vi "Periodic Tasks.vi"(8 "error in":errorcluster) -> ()   [LabVIEW 2017]
doc: "This VI runs in parallel to other tasks. It can contain as many user-defined periodic loops as you need. These can carry out PID or other sorts of timed response."
uses:
  HuskieBoard.ctl
  Log Queue.ctl
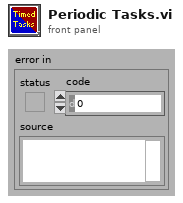
[diagram p1: front panel]
types:
  T1 = typedef "Log Queue.ctl" = enum16{"Log Queue"}
  T2 = typedef "HuskieBoard.ctl" = enum16{"HuskieBoard"}
  T3 = typedef "WPI_JoystickDevRef.ctl" = cluster{"Device":T4}
  T4 = typedef "WPI_JoystickDeviceEnum.ctl" = enum16{"USB 0", "USB 1", "USB 2", "USB 3", "USB 4", "USB 5"}
  T5 = typedef "WPI_RobotDriveDevRef.ctl" = cluster{"DevStatus":errorcluster, "Motors[]":T6[], "Square Inputs":bool, "Max Output":dbl}
  T6 = typedef "WPI_MotorControlDeviceRef.ctl" = cluster{"DeviceStatus":errorcluster, "Type":T7, "PWM":cluster{"PWM Channel":T8, "DeadBand":T9}, "CAN":cluster{"Device Number":u8, "SetOutput VI Ref":variant, "GetOutput VI Ref":variant, "Enable VI Ref":variant, "Disable VI Ref":variant, "Data":variant}, "Invert":bool, "DIO PWM":cluster{"PWM \"Enable\" Channel":T8, "DIOChannel":T10, "PWM Rate":dbl}}
  T7 = typedef "WPI_MotorControlType.ctl" = enum16{"PWM", "CAN", "DIO PWM"}
  T8 = typedef "FPGA_DIOPWMChannel.ctl" = enum8{"PWM 0", "PWM 1", "PWM 2", "PWM 3", "PWM 4", "PWM 5", "PWM 6", "PWM 7", "PWM 8", "PWM 9", "PWM MXP 0", "PWM MXP 1", "PWM MXP 2", "PWM MXP 3", "PWM MXP 4", "PWM MXP 5", "PWM MXP 6", "PWM MXP 7", "PWM MXP 8", "PWM MXP 9", "Invalid"}
  T9 = typedef "WPI_PWMDeadband.ctl" = cluster{"Name":string, "maxPositivePwm":i32, "minPositivePwm":i32, "centerPwm":i32, "maxNegativePwm":i32, "minNegativePwm":i32, "angularRange":u16}
  T10 = typedef "FPGA_DIOChannel.ctl" = enum8{"DIO 0", "DIO 1", "DIO 2", "DIO 3", "DIO 4", "DIO 5", "DIO 6", "DIO 7", "DIO 8", "DIO 9", "DIO MXP 0", "DIO MXP 1", "DIO MXP 2", "DIO MXP 3", "DIO MXP 4", "DIO MXP 5", "DIO MXP 6", "DIO MXP 7", "DIO MXP 8", "DIO MXP 9", "DIO MXP 10", "DIO MXP 11", "DIO MXP 12", "DIO MXP 13", "DIO MXP 14", "DIO MXP 15", "SPI Port CS1", "SPI Port CS2", "SPI Port CS3", "SPI Port MISO", "SPI Port MOSI", "Invalid"}
  T11 = cluster{"JoystickDevRef":T3, "RobotDriveDevRef":T5}
  T12 = typedef "WPI_SerialPortRef.ctl" = cluster{"DevStatus":errorcluster, "Serial Port Name":refnum<visa-resource-name>}
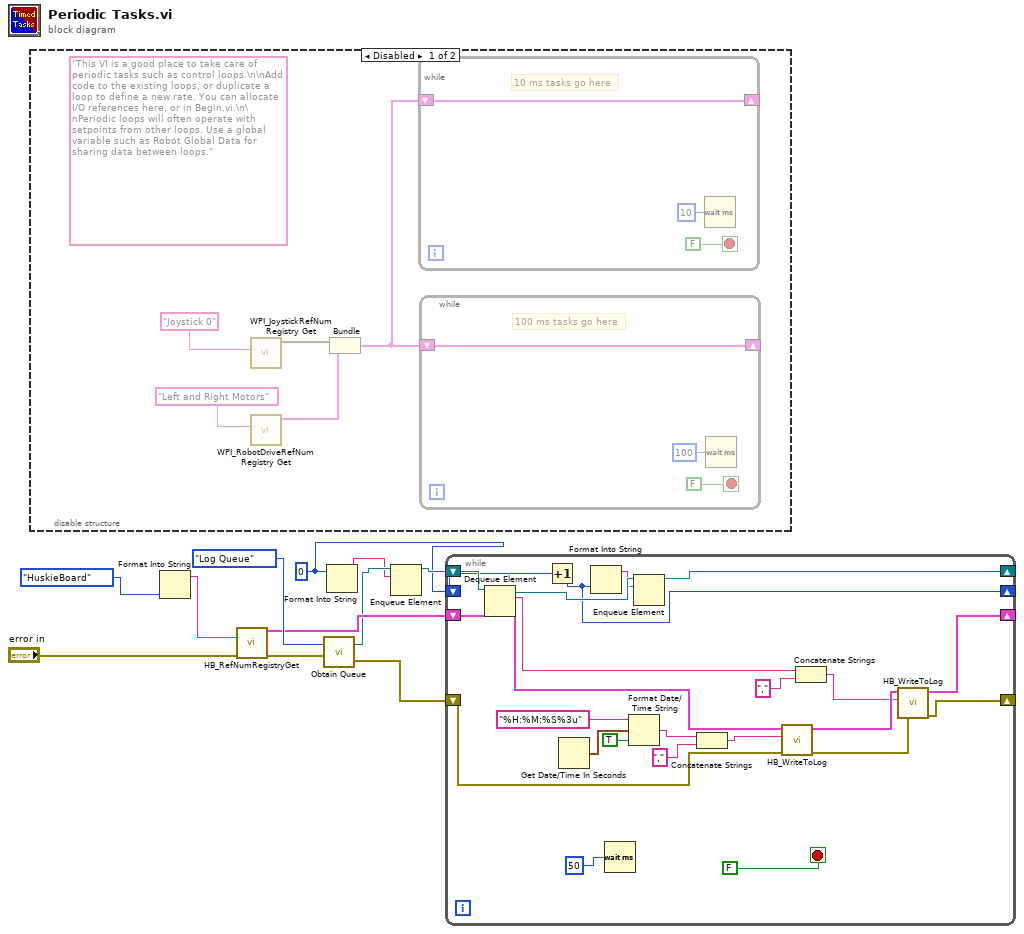
[diagram p0: block diagram]
diagram:
  w1 = 0
  n1 = disable-structure shown="Disabled" {
    frame Disabled {
      (unwired) "This VI is a good place to take care of periodic tasks such as control loops.\n\nAdd code to the existing loops, or duplicate a loop to define a new rate. You can allocate I/O references here, or in Begin.vi.\n\nPeriodic loops will often operate with setpoints from other loops. Use a global variable such as Robot Global Data for sharing data between loops."
      n2 = call <vilib>:"WPI_JoystickRefNum Registry Get.vi"("refnum name"="Joystick 0") -> ("JoystickDevRef"=w14:T3)  [unwired: 1 in, 9 out]
      n3 = call <vilib>:"WPI_RobotDriveRefNum Registry Get.vi"("refnum name"="Left and Right Motors") -> ("RobotDriveDevRef"=w13:T5)  [unwired: 1 in, 9 out]
      n4 = Bundle("JoystickDevRef"=w14, "RobotDriveDevRef"=w13) -> (w12:T11)  [unwired: 1 out]
      n5 = while {
        shift-right: [w20] -> _
        shift-left: w12 -> [w20]
        stop <- FALSE stop-if-true
        # "10 ms tasks go here"
        n6 = Wait (ms)(milliseconds to wait=u32 10) -> ()  [unwired: 1 out]
      }
      n7 = while {
        shift-right: [w17] -> _
        shift-left: w12 -> [w17]
        stop <- FALSE stop-if-true
        # "100 ms tasks go here"
        n8 = Wait (ms)(milliseconds to wait=u32 100) -> ()  [unwired: 1 out]
      }
    }
    frame Enabled {
    }
  }
  n9 = Format Into String(HuskieBoard."HuskieBoard" ("Enum")) -> (resulting string=w10:string)  [unwired: 3 in, 1 out]
  n10 = call <vilib>:"HB_RefNumRegistryGet.vi"("refnum name"=w10, "error in (no error)"="error in") -> ("HBDevRef"=w5:T12, "error out"=w7:errorcluster)  [unwired: 12 in]
  n11 = call "Obtain Queue.vi"("error in"=w7, "Queue"=Log_Queue."Log Queue" ("Enum")) -> ("error out"=w6:errorcluster, "Queue Ref"=w4:refnum<queue>)
  n12 = Format Into String(w1) -> (resulting string=w3:string)  [unwired: 3 in, 1 out]
  n13 = Enqueue Element(queue=w4, element=w3) -> (queue out=w2:refnum<queue>)  [unwired: 2 in, 2 out]
  n14 = while {
    shift-right: [w43] -> _
    shift-left: w5 -> [w31]
    shift-right: [w29] -> _
    shift-left: w6 -> [w36]
    shift-right: [w38] -> _
    shift-left: w2 -> [w42]
    shift-right: [w37] -> _
    shift-left: w1 -> [w41]
    stop <- FALSE stop-if-true
    n15 = Dequeue Element(queue=w42) -> (queue out=w40:refnum<queue>, element=w25:string)  [unwired: 2 in, 2 out]
    n16 = Increment(x=w41) -> (x+1=w37:i32)
    n17 = Get Date/Time In Seconds() -> (seconds since 1Jan1904=w34:timestamp)
    n18 = Format Into String(w37) -> (resulting string=w39:string)  [unwired: 3 in, 1 out]
    n19 = Wait (ms)(milliseconds to wait=u32 50) -> ()  [unwired: 1 out]
    n20 = Format Date/Time String(time format string (%c)="%H:%M:%S%3u", seconds (now)=w34, UTC format=TRUE) -> (date/time string=w28:string)
    n21 = Enqueue Element(queue=w40, element=w39) -> (queue out=w38:refnum<queue>)  [unwired: 2 in, 2 out]
    n22 = Concatenate Strings(w28, ",") -> (w27:string)
    n23 = call <vilib>:"HB_WriteToLog.vi"("error in (no error)"=w36, "Log string"=w27, "HBDevRef"=w31) -> ("error out"=w35:errorcluster, "HBDevRef"=w30:T12)  [unwired: 7 in]
    n24 = Concatenate Strings(w25, ",") -> (w23:string)
    n25 = call <vilib>:"HB_WriteToLog.vi"("error in (no error)"=w35, "Log string"=w23, "HBDevRef"=w30) -> ("error out"=w29:errorcluster, "HBDevRef"=w43:T12)  [unwired: 7 in]
  }
